vi "Test Get In ProgramFiles.vi"() -> ()   [LabVIEW 2021, in "Path Utilities.lvlib"]
doc: "Unit Test for \"Get In ProgramFiles.vi\"."
uses:
  Path Utilities.lvlib
panel:
  out "error out":errorcluster
  out "Pass - System Path with Base":bool
  out "Result - System Path with Base":path
  out "Expected - System Path with Base":path
  out "Pass - System Path Only":bool
  out "Result - System Path Only":path
  out "Expected - System Path Only":path
  in  "Base Path":path=path "Company/Application"
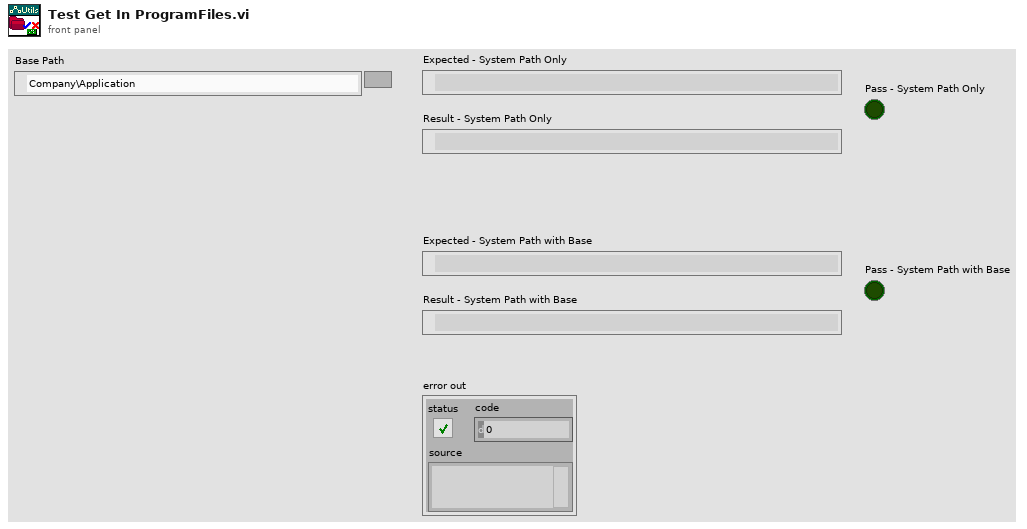
[diagram p1: front panel]
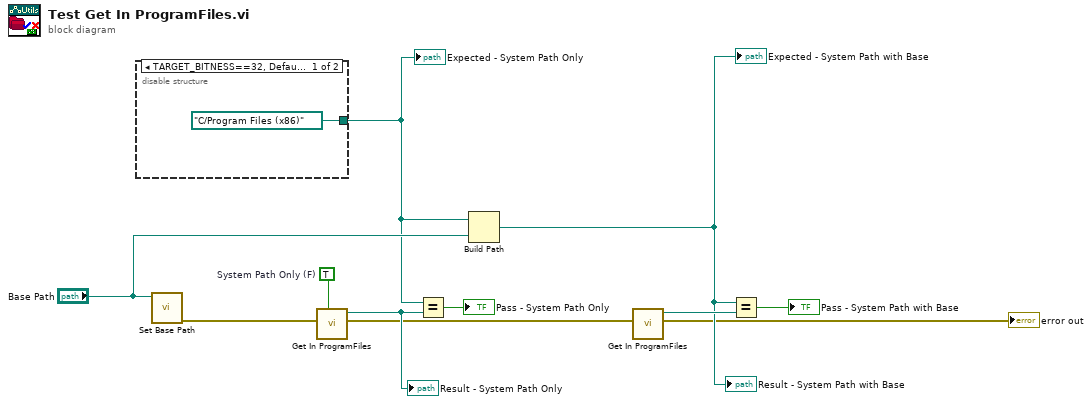
[diagram p0: block diagram]
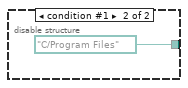
[diagram p2: hidden frame]
diagram:
  w10 = TRUE  # System Path Only (F)
  n1 = disable-structure shown="TARGET_BITNESS==32, Default" {
    disable-tunnel: [path "C:/Program Files (x86)" path "C:/Program Files"] -> w5
    frame condition #0 (active) {
    }
    frame condition #1 {
    }
  }
  "Expected - System Path Only" <- w5
  n2 = call "Set Base Path.vi"("Base Path"="Base Path") -> ("error out"=w11:errorcluster)  [unwired: 9 in, 1 out]
  n3 = call "Get In ProgramFiles.vi"("System Path Only (F)"=w10, "error in (no error)"=w11) -> ("error out"=w7:errorcluster, "Path"=w8:path)  [unwired: 8 in]
  "Result - System Path Only" <- w8
  n4 = Equal?(x=w5, y=w8) -> (x = y?=→"Pass - System Path Only":bool)
  n5 = Build Path(base path=w5, name or relative path="Base Path") -> (appended path=w2:path)
  "Expected - System Path with Base" <- w2
  "Result - System Path with Base" <- w2
  n6 = call "Get In ProgramFiles.vi"("error in (no error)"=w7) -> ("error out"=→"error out":errorcluster, "Path"=w4:path)  [unwired: 9 in]
  n7 = Equal?(x=w2, y=w4) -> (x = y?=→"Pass - System Path with Base":bool)
